vi "RDB Init.vi"(8 "error in":errorcluster, 11 "Compiled.Settings":T8={"Name"="", "RDB Data Receive "=[], "RDB Data Sent"=[], "vclient"=path "", "Network Settings"={"IP adress"="127.0.0.1", "RDB"={"Protocol"=enum."UDP", "Tx Port"=48270, "Rx Port"=10, "Buffer Size"=204800, "Timeout"=10}, "SCP"={"Protocol"=enum."TCP", "Tx Port"=48191, "Rx Port"=48191, "Buffer Size"=204800, "Timeout"=10}}, "SensorInfos"=[], "mmanager"=path "", "Scenario Paths"=[], "Custom SCP Commands"=[], "Timed Loop Settings for TaskControl"={"Period(ms)"=2, "Priority"=100, "Processor"=-2}, "Timed Loop Settings for ModuleManager"={"Period(ms)"=2, "Priority"=100, "Processor"=-2}}) -> (0 "error out":errorcluster, 2 "RDB References":T4 {"RDB Send Reference"."RDB Data"."payload" format="%x"; "RDB Send Reference"."RDB Data"."timestamp" format="%<%.7X\n%x>T"; "RDB Send Reference"."RDB Data"."type" items=["FlexRay Data"=32, "FlexRay Null"=33, "FlexRay Symbol"=34, "Log Trigger"=225, "Start Trigger"=226]; "RDB Send Reference"."RDB Data"."cycle count" max=63 step=1; "RDB Receive Reference"."RDB Data"."payload" format="%x"; "RDB Receive Reference"."RDB Data"."timestamp" format="%<%.7X\n%x>T"; "RDB Receive Reference"."RDB Data"."type" items=["FlexRay Data"=32, "FlexRay Null"=33, "FlexRay Symbol"=34, "Log Trigger"=225, "Start Trigger"=226]; "RDB Receive Reference"."RDB Data"."cycle count" max=63 step=1}, 3 "Settings":T1={"UDP Receiver"=refnum, "UDP Sender"=refnum, "Valid Packet"=FALSE, "TCP"=refnum, "Network Settings"={"IP adress"="127.0.0.1", "RDB"={"Protocol"=enum."UDP", "Tx Port"=48191, "Rx Port"=48191, "Buffer Size"=204800, "Timeout"=10}, "SCP"={"Protocol"=enum."TCP", "Tx Port"=48191, "Rx Port"=48191, "Buffer Size"=204800, "Timeout"=10}}, "vclient"=path "", "paeseHandle"=0})   [LabVIEW 2023, in "RDB.lvlib"]
uses:
  RDB.lvlib
  Shared/Compiled.Settings.ctl
  System Explorer/RDB Data.ctl
  RDB Object.ctl
  RDB Player Object.ctl
  Shared/Network Settings.ctl
  Shared/Protocol.ctl
  Shared/SensorInfos.ctl
  Shared/SensorInfo.ctl
  Shared/Sensor Name.ctl
  MM/MM Data.ctl
  MM/MM Objects.ctl
  MM/MM Object.ctl
  Shared/Timedloop Settings.ctl
  RDB References.ctl
  RDB Reference.ctl
  <vilib>/xnet/xnet.llb/XNET Frame FlexRay.ctl
  <vilib>/xnet/xnet.llb/XNET Frame Type FlexRay.ctl
  Engine/Type/Settings.ctl
  Shared/Vires VTD Shared.lvlib
  Engine/Vires VTD Engine.lvlib
  MM/MM.lvlib
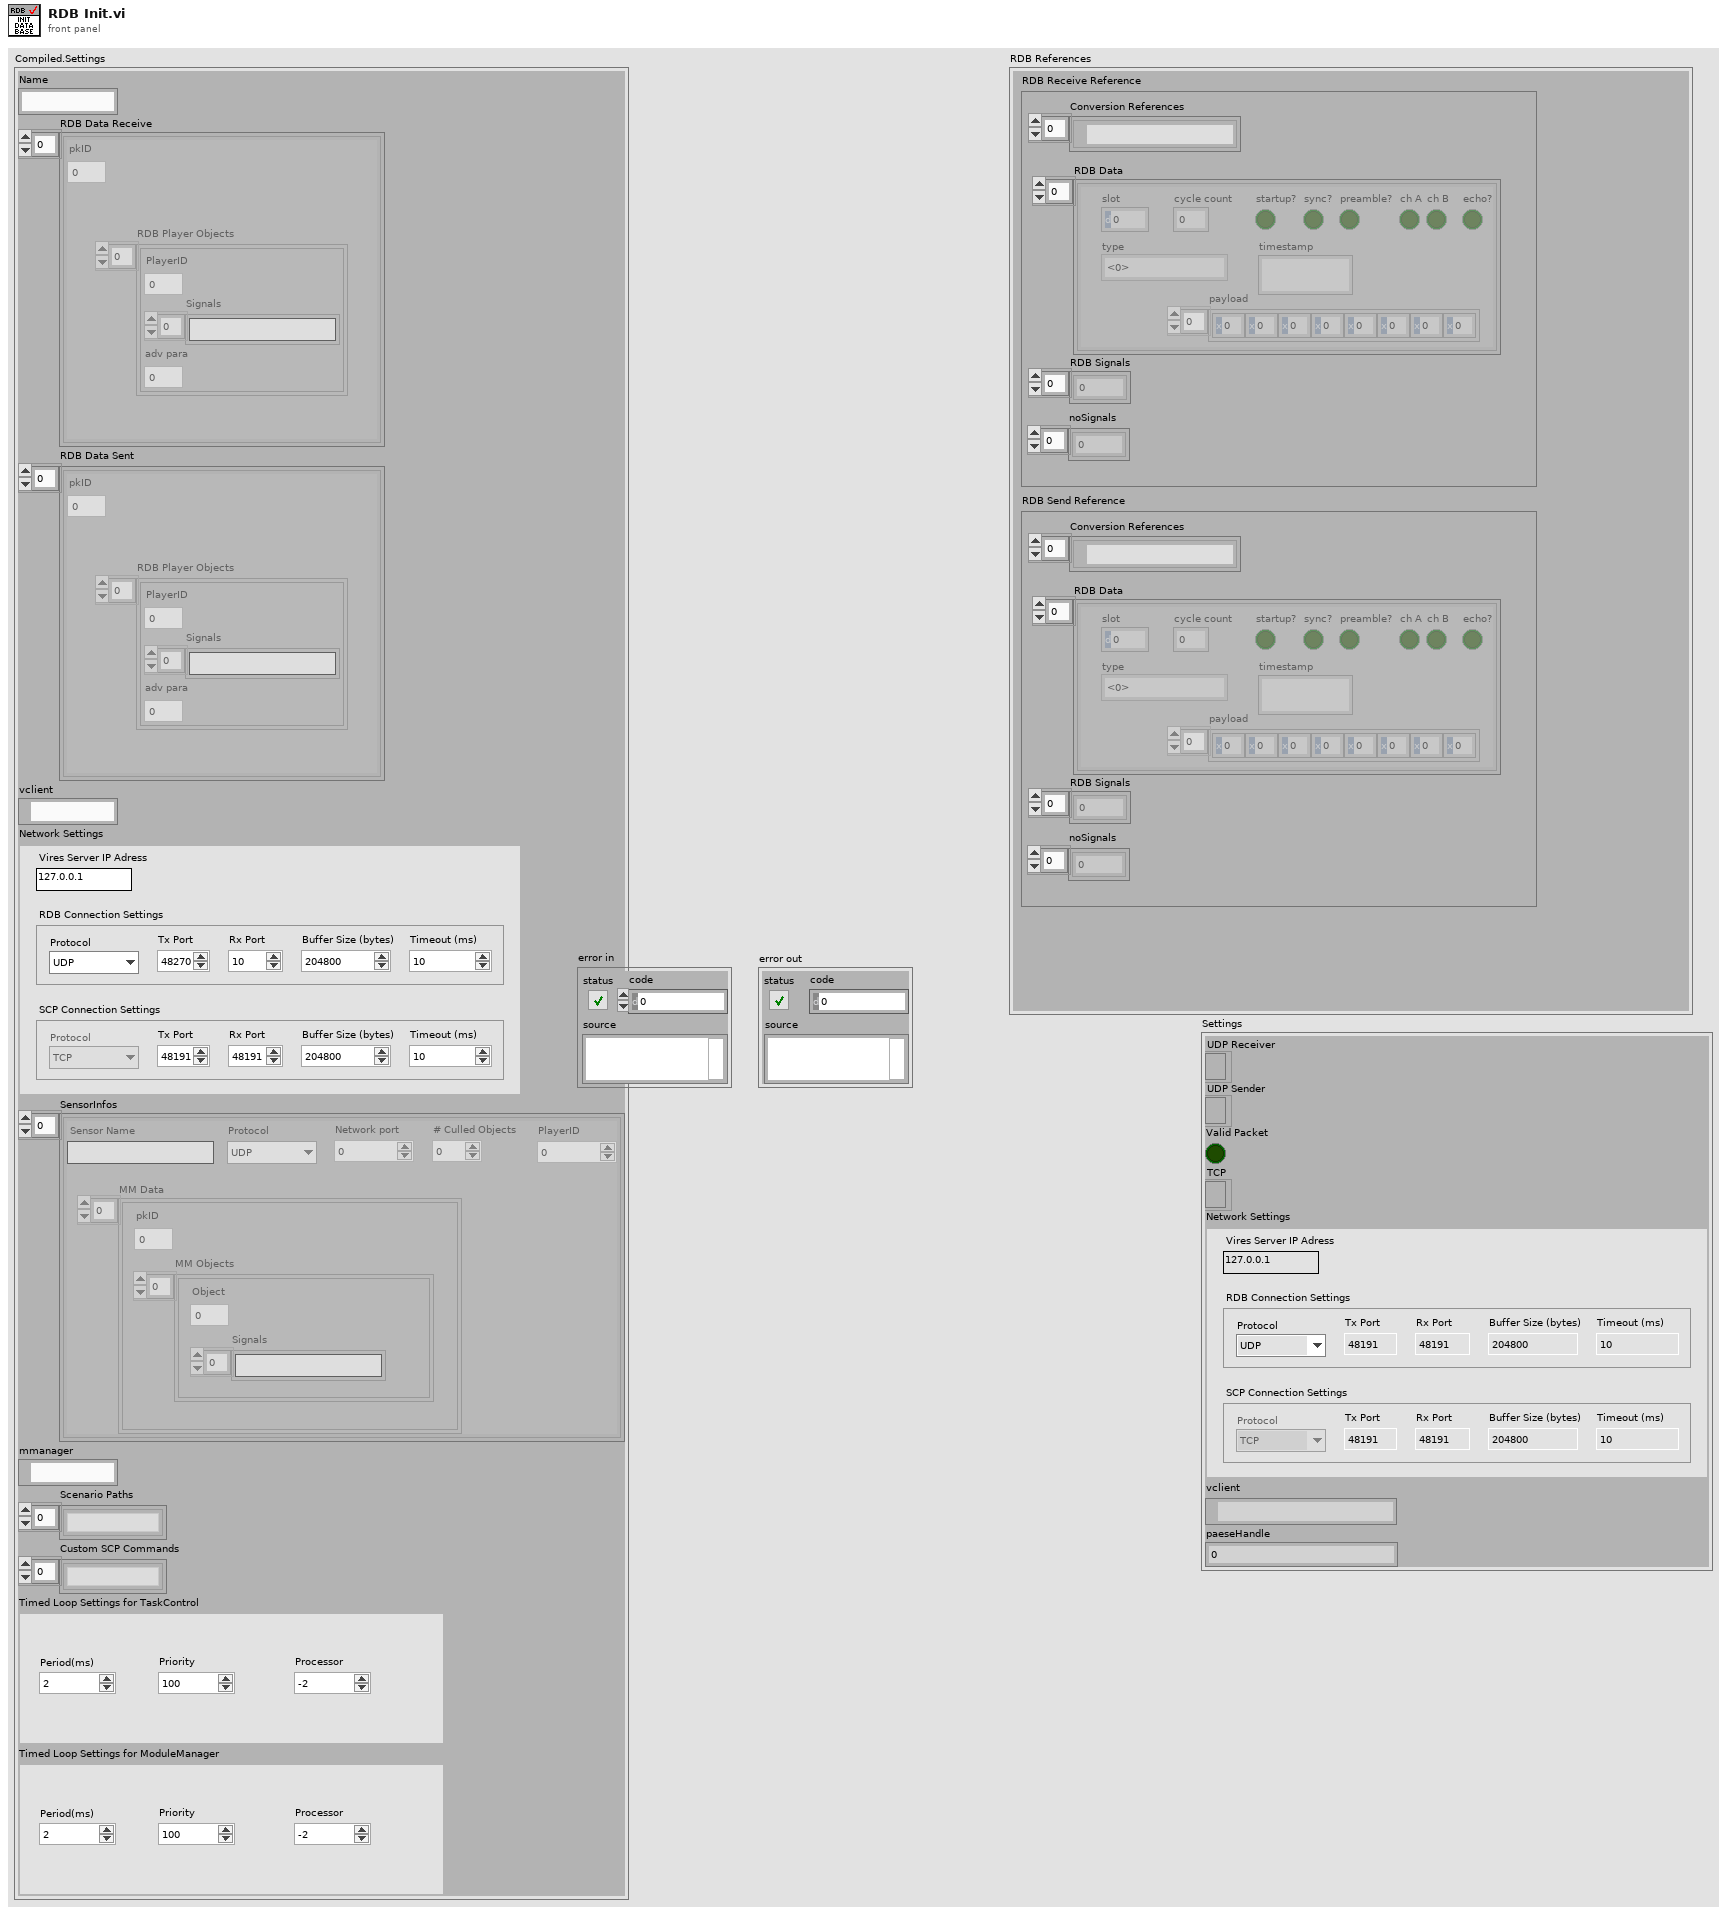
[diagram p1: front panel]
types:
  T1 = typedef "Vires VTD Engine.lvlib/Settings.ctl" = cluster{"UDP Receiver":refnum<k16>, "UDP Sender":refnum<k16>, "Valid Packet":bool, "TCP":refnum<k5>, "Network Settings":T2, "vclient":path, "paeseHandle":u64}
  T2 = typedef "Vires VTD Shared.lvlib/Network Settings.ctl" = cluster{"IP adress":string, "RDB":cluster{"Protocol":T3, "Tx Port":u16, "Rx Port":u16, "Buffer Size":i32, "Timeout":u16}, "SCP":cluster{"Protocol":T3, "Tx Port":u16, "Rx Port":u16, "Buffer Size":i32, "Timeout":u16}}
  T3 = typedef "Vires VTD Shared.lvlib/Protocol.ctl" = enum16{"UDP", "TCP"}
  T4 = typedef "RDB.lvlib/RDB References.ctl" = cluster{"RDB Receive Reference":T5, "RDB Send Reference":T5}
  T5 = typedef "RDB.lvlib/RDB Reference.ctl" = cluster{"Conversion References":refnum<k21>[], "RDB Data":T6[], "RDB Signals":dbl[], "noSignals":i32[]}
  T6 = typedef "XNET Frame FlexRay.ctl" = cluster{"timestamp":timestamp, "payload":u8[], "slot":u16, "type":T7, "cycle count":u8, "startup?":bool, "sync?":bool, "preamble?":bool, "ch A":bool, "ch B":bool, "echo?":bool}
  T7 = typedef "XNET Frame Type FlexRay.ctl" = u8
  T8 = typedef "Vires VTD Shared.lvlib/Compiled.Settings.ctl" = cluster{"Name":string, "RDB Data Receive ":T9, "RDB Data Sent":T9, "vclient":path, "Network Settings":T2, "SensorInfos":T12, "mmanager":path, "Scenario Paths":string[], "Custom SCP Commands":string[], "Timed Loop Settings for TaskControl":T18, "Timed Loop Settings for ModuleManager":T18}
  T9 = typedef "Vires VTD Shared.lvlib/RDB Data.ctl" = T10[]
  T10 = typedef "RDB.lvlib/RDB Object.ctl" = cluster{"pkID":i32, "RDB Player Objects":T11[]}
  T11 = typedef "RDB.lvlib/RDB Player Object.ctl" = cluster{"PlayerID":i32, "Signals":string[], "adv para":i32}
  T12 = typedef "Vires VTD Shared.lvlib/SensorInfos.ctl" = T13[]
  T13 = typedef "Vires VTD Shared.lvlib/SensorInfo.ctl" = cluster{"Sensor Name":T14, "Protocol":T3, "Network port":i32, "# Culled Objects":i32, "PlayerID":u8, "MM Data":T15}
  T14 = typedef "Vires VTD Shared.lvlib/Sensor Name.ctl" = string
  T15 = typedef "Vires VTD Shared.lvlib/MM Data.ctl" = T16[]
  T16 = typedef "MM.lvlib/MM Objects.ctl" = cluster{"pkID":i32, "MM Objects":T17[]}
  T17 = typedef "MM.lvlib/MM Object.ctl" = cluster{"Object":i32, "Signals":string[]}
  T18 = typedef "Vires VTD Shared.lvlib/Timedloop Settings.ctl" = cluster{"Period(ms)":i64, "Priority":i32, "Processor":i32}
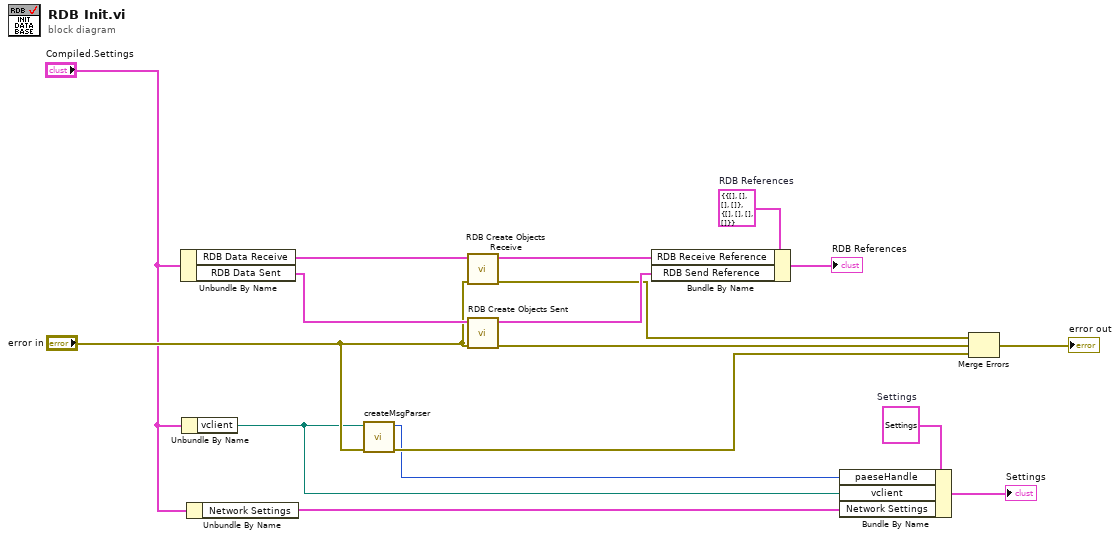
[diagram p0: block diagram]
diagram:
  w5 = T1 {"UDP Receiver"=refnum, "UDP Sender"=refnum, "Valid Packet"=FALSE, "TCP"=refnum, "Network Settings"={"IP adress"="127.0.0.1", "RDB"={"Protocol"=enum."UDP", "Tx Port"=48270, "Rx Port"=10, "Buffer Size"=204800, "Timeout"=10}, "SCP"={"Protocol"=enum."TCP", "Tx Port"=48191, "Rx Port"=48191, "Buffer Size"=204800, "Timeout"=10}}, "vclient"=path "", "paeseHandle"=0}  # Settings
  w17 = T4 {"RDB Receive Reference"={"Conversion References"=[], "RDB Data"=[], "RDB Signals"=[], "noSignals"=[]}, "RDB Send Reference"={"Conversion References"=[], "RDB Data"=[], "RDB Signals"=[], "noSignals"=[]}}  # RDB References
  n1 = Unbundle By Name("Compiled.Settings") -> ("RDB Data Receive"=w15:T9, "RDB Data Sent"=w14:T9)
  n2 = Unbundle By Name("Compiled.Settings") -> ("vclient"=w1:path)
  n3 = Unbundle By Name("Compiled.Settings") -> ("Network Settings"=w6:T2)
  n4 = call "createMsgParser.vi"("error in (no error)"="error in", "path in"=w1) -> ("error out"=w8:errorcluster, "paeseHandle"=w3:u64)  [unwired: 8 in]
  n5 = call "RDB Create Objects Receive.vi"("error in (no error)"="error in", "RDB Data Receive"=w15) -> ("error out"=w12:errorcluster, "RDB Reference"=w16:T5)  [unwired: 8 in]
  n6 = call "RDB Create Objects Sent.vi"("error in (no error)"="error in", "RDB Data Sent"=w14) -> ("error out"=w11:errorcluster, "RDB Reference"=w13:T5)  [unwired: 8 in]
  n7 = Bundle By Name(cluster=w17, "RDB Receive Reference"=w16, "RDB Send Reference"=w13) -> (→"RDB References":T4)
  n8 = Bundle By Name(cluster=w5, "paeseHandle"=w3, "vclient"=w1, "Network Settings"=w6) -> (→"Settings":T1)
  n9 = Merge Errors(w12, w11, w8) -> (→"error out":errorcluster)
